vi "Fdx Create Session (RX-Monitor).vi"(6 "PortMap":u32, 7 "MonitorConfig":T1 {"DefaultCronoMode" items=["FDX_RX_DEFAULT_ENA_CNT", "FDX_RX_DEFAULT_MON_ENA_ALL", "FDX_RX_DEFAULT_MON_ENA_GOOD"]}, 8 "error in (no error)":errorcluster, 9 "DefaultPayloadMode (Full)":u32(ring) items=["FDX_PAYLOAD_FULL", "FDX_PAYLOAD_IP_EXT", "FDX_PAYLOAD_IP", "FDX_PAYLOAD_MAC"], 10 "port":u32, 11 "board":u32) -> (0 "error out":errorcluster, 1 "GlbMonBufferSizeOut":u32, 2 "PortInitOut":T2 {"PortConfig" items=["FDX_SINGLE", "FDX_REDUNDANT"]}, 3 "InstrumentHandle_port out":u32, 4 "Duplicated":bool, 5 "InstrumentHandle_board out":u32)   [LabVIEW 2020, in "AIM664LV.lvlib"]
uses:
  AIM664LV.lvlib
  _controls/session_monitor_config.ctl
  _controls/hwEntry_actions.ctl
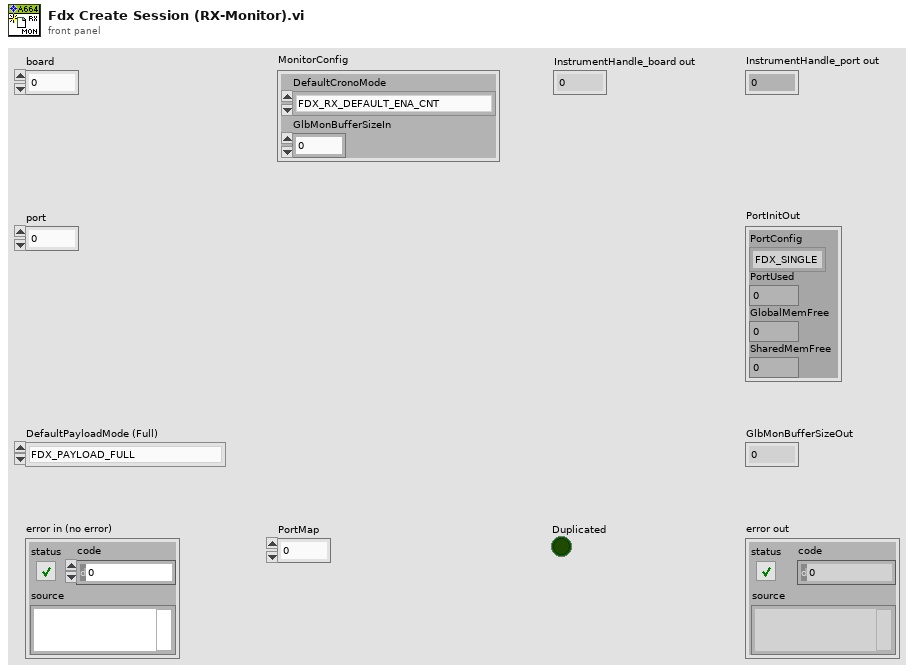
[diagram p1: front panel]
types:
  T1 = typedef "AIM664LV.lvlib/session_monitor_config.ctl" = cluster{"DefaultCronoMode":u32, "GlbMonBufferSizeIn":u32}
  T2 = cluster{"PortConfig":u32, "PortUsed":u32, "GlobalMemFree":u32, "SharedMemFree":u32}
  T3 = typedef "AIM664LV.lvlib/hwEntry_actions.ctl" = enum16{"Init Port", "Init Board", "Relase Port", "Release Board"}
  T4 = typedef "AIM664LV.lvlib/hwEntry_handleValidityFlag.ctl" = cluster{"boardHandleValid":bool, "portHandleValid":bool}
  T5 = cluster{"ReceiveMode":u32, "DefaultPayloadMode":u32, "DefaultCronoMode":u32, "GlbMonBufferSizeIn":u32, "RerosDefaultOutputPortmap":u32}
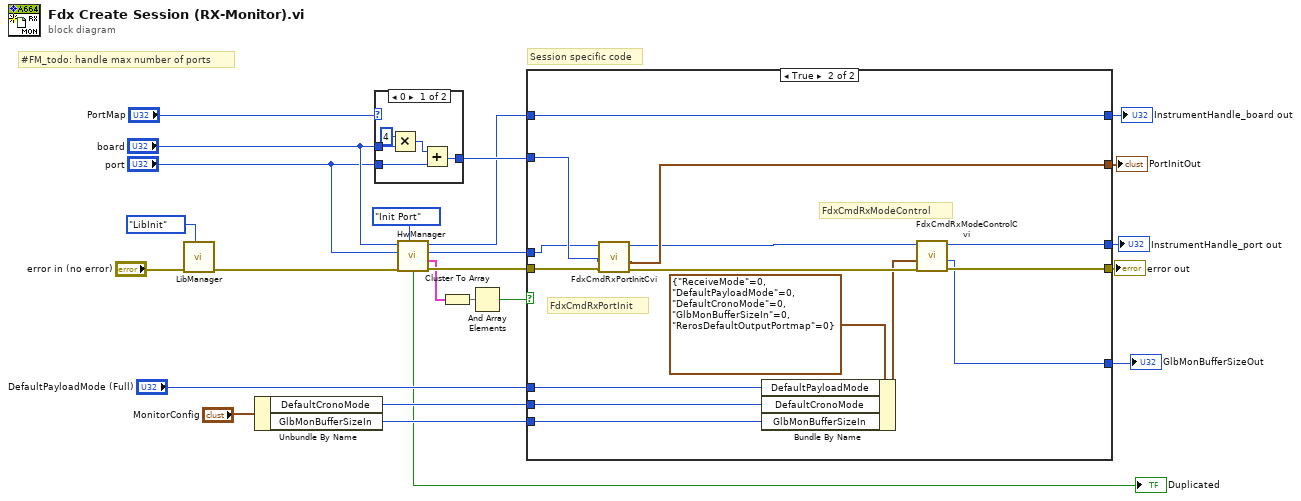
[diagram p0: block diagram]
diagram:
  # "Session specific code"
  # "#FM_todo: handle max number of ports"
  n1 = call "LibManager.vi"("action"=enum16{"LibInit", "LibExit"}."LibInit", "error in (no error)"="error in (no error)") -> ("error out"=w22:errorcluster)  [unwired: 7 in, 2 out]
  n2 = Unbundle By Name("MonitorConfig") -> ("DefaultCronoMode"=w10:u32, "GlbMonBufferSizeIn"=w9:u32)
  n3 = case shown="0" "PortMap" {
    selector: "PortMap" -> [_ w30]
    tunnel: "board" -> [w28 _]
    tunnel: "port" -> [w29 _]
    tunnel: [w25 w30] -> w14
    frame 0 {
      n4 = Multiply(x=u32 4, y=w28) -> (x*y=w26:u32)
      n5 = Add(x=w26, y=w29) -> (x+y=w25:u32)
    }
    frame Default {
    }
  }
  n6 = call "HwManager.vi"("action (Init)"=hwEntry_actions."Init Port", "error in (no error)"=w22, "port"="port", "board"="board") -> ("error out"=w21:errorcluster, "validityFlag"=w3:T4, "InstrumentHandle_port out"=w8:u32, "InstrumentHandle_board out"=w7:u32, "Duplicated"=→"Duplicated":bool)  [unwired: 3 in]
  n7 = Cluster To Array(cluster=w3) -> (array=w2:bool[])
  n8 = And Array Elements(Boolean array=w2) -> (logical AND=w1:bool)
  n9 = case shown="True" w1 {
    tunnel: w21 -> [w31 w46]
    tunnel: w8 -> [_ w44]
    tunnel: [w31 w40] -> w20
    tunnel: w14 -> [_ w45]
    tunnel: [_ w43] -> w19
    tunnel: w7 -> [_ w32]
    tunnel: [_ w33] -> w18
    tunnel: "DefaultPayloadMode (Full)" -> [_ w37]
    tunnel: [_ w36] -> w12
    tunnel: w10 -> [_ w35]
    tunnel: w9 -> [_ w34]
    tunnel: [_ w32] -> w4
    frame False {
    }
    frame True {
      # "FdxCmdRxModeControl"
      # "FdxCmdRxPortInit"
      n10 = call "FdxCmdRxPortInitCvi.vi"("error in"=w46, "PortMap"=w45, "InstrumentHandle_port"=w44) -> ("error out"=w42:errorcluster, "PortInitOut"=w43:T2, "InstrumentHandle_port"=w41:u32)  [unwired: 6 in]
      n11 = Bundle By Name(cluster=T5 {"ReceiveMode"=0, "DefaultPayloadMode"=0, "DefaultCronoMode"=0, "GlbMonBufferSizeIn"=0, "RerosDefaultOutputPortmap"=0} ("RxModeControlIn"), "DefaultPayloadMode"=w37, "DefaultCronoMode"=w35, "GlbMonBufferSizeIn"=w34) -> (w38:T5)
      n12 = call "FdxCmdRxModeControlCvi.vi"("error in"=w42, "RxModeControlIn"=w38, "InstrumentHandle_port"=w41) -> ("error out"=w40:errorcluster, "GlbMonBufferSizeOut"=w36:u32, "InstrumentHandle_port"=w33:u32)  [unwired: 6 in]
    }
  }
  "error out" <- w20
  "PortInitOut" <- w19
  "InstrumentHandle_port out" <- w18
  "GlbMonBufferSizeOut" <- w12
  "InstrumentHandle_board out" <- w4
